vi "Create Process.vi"(5 "use stderr (F)":bool, 7 "hide window (T)":bool=TRUE, 8 "error in":errorcluster, 9 "dir or path to lv_proc.dll (.)":path, 10 "command":string, 11 "working directory":string) -> (0 "error out":errorcluster, 3 "pipe out":T1)   [LabVIEW 2018, in "LV Process library.lvlib"]
doc: "Calls lv_proc.dll function to create a new process and return pipe handle. Process is started by 'command' in 'working directory', and window is hidden if selected. Standard error pipe can be used. If directory with lv_proc.dll or path to lv_proc.dll is not specified, current application directory is used.\n\nEven if the process instance has returned exit code (i.e. process finished) the handle must be closed by proc_cleanup.vi.\n\n---\nLV Process works only with lv_proc.dll library, which is part of vipm package or should be delivered together with packed library. Placement of this dll is selected in terminal of Create Process.vi."
uses:
  LV Process library.lvlib
  Pipe Handle.ctl
  <vilib>/Utility/error.llb/Error Cluster From Error Code.vi
  <vilib>/ErrorRing/Error Ring.xnode
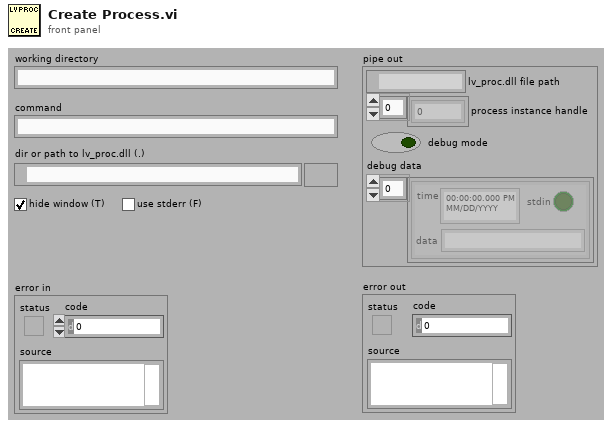
[diagram p1: front panel]
types:
  T1 = typedef "LV Process library.lvlib/Pipe Handle.ctl" = cluster{"lv_proc.dll file path":path, "process instance handle":u32[], "debug mode":bool, "debug data":cluster{"time":timestamp, "stdin":bool, "data":string}[]}
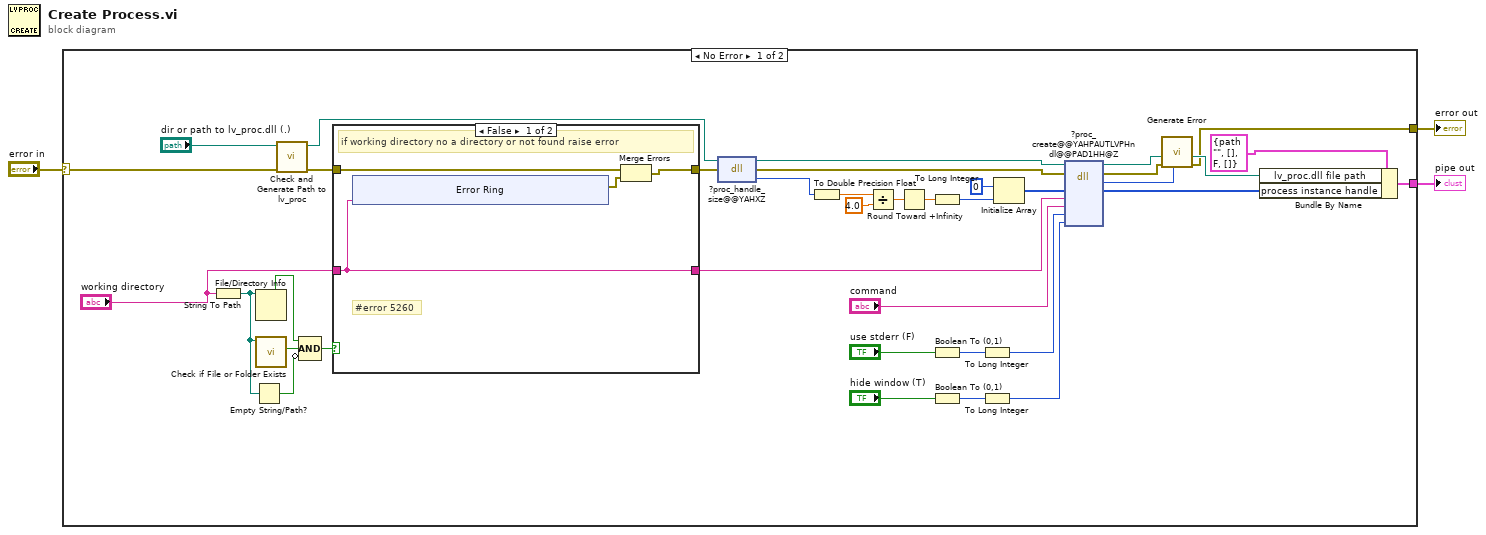
[diagram p0: block diagram]
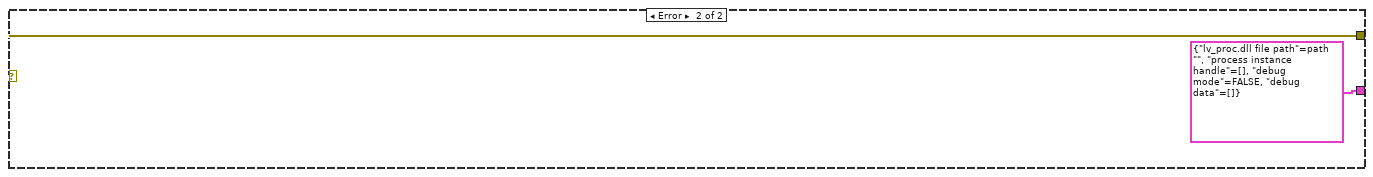
[diagram p3: hidden frame]
diagram:
  n1 = case shown="No Error" "error in" {
    selector: "error in" -> [w6 w55]
    tunnel: [w21 w55] -> w2
    tunnel: [w27 T1 {"lv_proc.dll file path"=path "", "process instance handle"=[], "debug mode"=FALSE, "debug data"=[]} ("pipe handle out")] -> w1
    frame No Error {
      n2 = String To Path(string="working directory") -> (path=w5:path)
      n3 = Empty String/Path?(string/path=w5) -> (empty?=w4:bool)
      n4 = File/Directory Info(path=w5) -> (directory=w13:bool)  [unwired: 1 in, 6 out]
      n5 = call <vilib>:"Check if File or Folder Exists.vi"("path"=w5) -> ("file or folder exists?"=w12:bool)  [unwired: 8 in, 2 out]
      n6 = call "Check and Generate Path to lv_proc.vi"("error in (no error)"=w6, "dir or path to lv_proc.dll (.)"="dir or path to lv_proc.dll (.)") -> ("error out"=w8:errorcluster, "dup path"=w29:path)  [unwired: 8 in]
      n7 = Compound Arithmetic op=AND(w13, w12, invert w4) -> (w11:bool)
      n8 = case shown="False" w11 {
        tunnel: "working directory" -> [w44 w52]
        tunnel: [w44 w52] -> w9
        tunnel: w8 -> [w42 w53]
        tunnel: [w41 w53] -> w7
        frame False {
          # "#error 5260"
          # "if working directory no a directory or not found raise error"
          n9 = xnode "Error Ring"("parameter 0"=w44) -> ("error out"=w43:errorcluster)
          n10 = Merge Errors(w42, w43) -> (w41:errorcluster)
        }
        frame True {
        }
      }
      n11 = dll-call lib="C:/Data/GOLPI/LV Process/lv_proc.dll" fn="?proc_handle_size@@YAHXZ" label="proc_handle_size"(path in=w29, error in=w7) -> (path out=w30:path, error out=w31:errorcluster, "size [B]"=w17:i32)  [unwired: 1 in]
      n12 = To Double Precision Float(number=w17) -> (double precision float=w19:dbl)
      n13 = Divide(x=w19, y=4.0) -> (x/y=w16:dbl)
      n14 = Round Toward +Infinity(x=w16) -> (ceil(x): smallest int >= x=w15:dbl)
      n15 = To Long Integer(number=w15) -> (32bit integer=w18:i32)
      n16 = Boolean To (0,1)(Boolean="use stderr (F)") -> (0, 1=w35:i16)
      n17 = Boolean To (0,1)(Boolean="hide window (T)") -> (0, 1=w37:i16)
      n18 = To Long Integer(number=w35) -> (32bit integer=w34:i32)
      n19 = To Long Integer(number=w37) -> (32bit integer=w36:i32)
      n20 = Initialize Array(u32 0 ("element"), w18) -> (w32:u32[])
      n21 = dll-call lib="C:/Data/GOLPI/LV Process/lv_proc.dll" fn="?proc_create@@YAHPAUTLVPHndl@@PAD1HH@Z" label="proc_create"(path in=w30, error in=w31, "proc"=w32, "folder"=w9, "command"="command", "use_stderr"=w34, "hide_window"=w36) -> (path out=w24:path, error out=w23:errorcluster, "error"=w28:i32, "proc"=w25:u32[])  [unwired: 5 in]
      n22 = call "Generate Error.vi"("error code in"=w28, "error in"=w23, "lv_proc.dll path in"=w24) -> ("error out"=w21:errorcluster, "lv_proc.dll path out"=w22:path)  [unwired: 6 in]
      n23 = Bundle By Name(cluster=T1 {"lv_proc.dll file path"=path "", "process instance handle"=[], "debug mode"=FALSE, "debug data"=[]} ("pipe"), "lv_proc.dll file path"=w22, "process instance handle"=w25) -> (w27:T1)
    }
    frame Error {
    }
  }
  "error out" <- w2
  "pipe out" <- w1
